vi "CreateSampleDelayLookup.vi"(8 "error in":errorcluster, 10 "Last Dynamic Module":string) -> (0 "error out":errorcluster, 3 "lookup":variant)   [LabVIEW 2017, in "CmsAcquisition.lvlib"]
uses:
  <vilib>/addons/InsightCM/Devices/Shared/Cms/CmsAcquisition/CmsAcquisition.lvlib
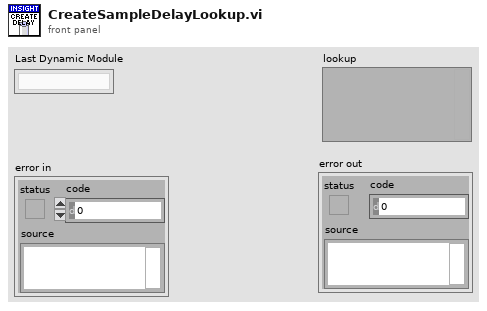
[diagram p1: front panel]
types:
  T1 = cluster{"Sampling Rate":i32, "Delay Compensation (samples)":dbl}[]
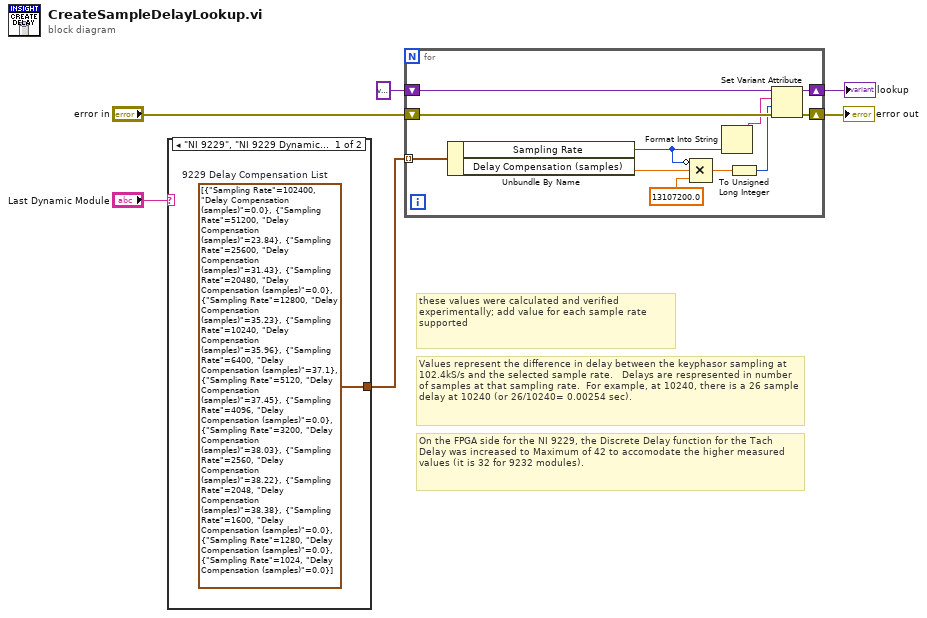
[diagram p0: block diagram]
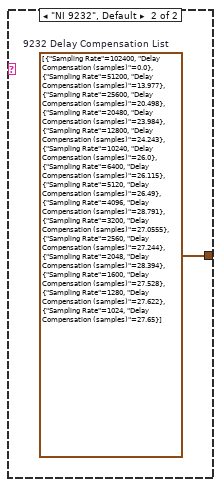
[diagram p2: hidden frame]
diagram:
  # "On the FPGA side for the NI 9229, the Discrete Delay function for the Tach Delay was increased to Maximum of 42 to accomodate the higher measured values (it is 32 for 9232 modules)."
  # "Values represent the difference in delay between the keyphasor sampling at 102.4kS/s and the selected sample rate.   Delays are respresented in number of samples at that sampling rate.  For example, at 10240, there is a 26 sample delay at 10240 (or 26/10240= 0.00254 sec)."
  # "these values were calculated and verified experimentally; add value for each sample rate supported"
  n1 = case shown="\"NI 9229\", \"NI 9229 Dynamic\"" "Last Dynamic Module" {
    tunnel: [w7 w8] -> w1
    frame "NI 9229", "NI 9229 Dynamic" {
      w7 = T1 [{"Sampling Rate"=102400, "Delay Compensation (samples)"=0.0}, {"Sampling Rate"=51200, "Delay Compensation (samples)"=23.84}, {"Sampling Rate"=25600, "Delay Compensation (samples)"=31.43}, {"Sampling Rate"=20480, "Delay Compensation (samples)"=0.0}, {"Sampling Rate"=12800, "Delay Compensation (samples)"=35.23}, {"Sampling Rate"=10240, "Delay Compensation (samples)"=35.96}, {"Sampling Rate"=6400, "Delay Compensation (samples)"=37.1}, {"Sampling Rate"=5120, "Delay Compensation (samples)"=37.45}, {"Sampling Rate"=4096, "Delay Compensation (samples)"=0.0}, {"Sampling Rate"=3200, "Delay Compensation (samples)"=38.03}, {"Sampling Rate"=2560, "Delay Compensation (samples)"=38.22}, {"Sampling Rate"=2048, "Delay Compensation (samples)"=38.38}, {"Sampling Rate"=1600, "Delay Compensation (samples)"=0.0}, {"Sampling Rate"=1280, "Delay Compensation (samples)"=0.0}, {"Sampling Rate"=1024, "Delay Compensation (samples)"=0.0}]  # 9229 Delay Compensation List
    }
    frame "NI 9232", Default {
      w8 = T1 [{"Sampling Rate"=102400, "Delay Compensation (samples)"=0.0}, {"Sampling Rate"=51200, "Delay Compensation (samples)"=13.977}, {"Sampling Rate"=25600, "Delay Compensation (samples)"=20.498}, {"Sampling Rate"=20480, "Delay Compensation (samples)"=23.984}, {"Sampling Rate"=12800, "Delay Compensation (samples)"=24.243}, {"Sampling Rate"=10240, "Delay Compensation (samples)"=26.0}, {"Sampling Rate"=6400, "Delay Compensation (samples)"=26.115}, {"Sampling Rate"=5120, "Delay Compensation (samples)"=26.49}, {"Sampling Rate"=4096, "Delay Compensation (samples)"=28.791}, {"Sampling Rate"=3200, "Delay Compensation (samples)"=27.0555}, {"Sampling Rate"=2560, "Delay Compensation (samples)"=27.244}, {"Sampling Rate"=2048, "Delay Compensation (samples)"=28.394}, {"Sampling Rate"=1600, "Delay Compensation (samples)"=27.528}, {"Sampling Rate"=1280, "Delay Compensation (samples)"=27.622}, {"Sampling Rate"=1024, "Delay Compensation (samples)"=27.65}]  # 9232 Delay Compensation List
    }
  }
  n2 = for {
    shift-right: [w18] -> w6
    shift-left: variant ("variant") -> [w19]
    shift-right: [w17] -> w4
    shift-left: "error in" -> [w16]
    tunnel: w1 -> [w13] mode=indexing
    n3 = Unbundle By Name(w13) -> ("Sampling Rate"=w10:i32, "Delay Compensation (samples)"=w11:dbl)
    n4 = Compound Arithmetic op=MULTIPLY(invert w10, w11, 13107200.0 ("SampClkTimebase")) -> (w15:dbl)
    n5 = Format Into String(w10) -> (resulting string=w9:string)  [unwired: 3 in, 1 out]
    n6 = To Unsigned Long Integer(number=w15) -> (unsigned 32bit integer=w12:u32)
    n7 = Set Variant Attribute(Variant=w19, name=w9, value=w12, error in=w16) -> (Variant out=w18:variant, error out=w17:errorcluster)  [unwired: 1 out]
  }
  "lookup" <- w6
  "error out" <- w4
